vi "RemoveNullTerminator.vi"(1 "inString":string) -> (0 "outString":string)   [LabVIEW 2012, in "Phidget Common.lvlib"]
uses:
  <instrlib>/Phidgets/Phidget Common/Phidget Common.lvlib
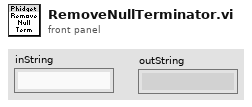
[diagram p1: front panel]
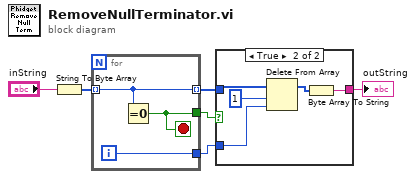
[diagram p0: block diagram]
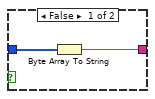
[diagram p2: hidden frame]
diagram:
  n1 = String To Byte Array(string="inString") -> (unsigned byte array=w6:u8[])
  n2 = for {
    tunnel: w6 -> [w9] mode=indexing
    tunnel: [w9] -> w5 mode=indexing
    tunnel: [w8] -> w4
    tunnel: [w7] -> w3
    i -> [w7]
    stop <- w8 stop-if-true
    n3 = Equal To 0?(x=w9) -> (x = 0?=w8:bool)
  }
  n4 = case shown="True" w4 {
    tunnel: [w11 w12] -> w1
    tunnel: w5 -> [w10 w16]
    tunnel: w3 -> [_ w15]
    frame False {
      n5 = Byte Array To String(unsigned byte array=w10) -> (string=w11:string)
    }
    frame True {
      n6 = Delete From Array(array=w16, length=1, index=w15) -> (array with subset deleted=w13:u8[])  [unwired: 1 out]
      n7 = Byte Array To String(unsigned byte array=w13) -> (string=w12:string)
    }
  }
  "outString" <- w1
